vi "CommonVIs_SpltStringIntoArguments.vi"(1 "String":string="\"1,2,3\",120,\"pelle,12\"", 3 "AddEmptyValues(False)":bool, 5 "error in (no error)":errorcluster) -> (15 "splittedString":string[](array[string]), 19 "error out":errorcluster)   [LabVIEW 2020]
doc: "SubVI to a <B>ScriptText</B> object.\n\n[GOOP 1.0]"
panel:
  # "\"1,2,3\",120,\"pelle,12\""
  # "pelle,12"
  # "1,2,3"
  # "120"
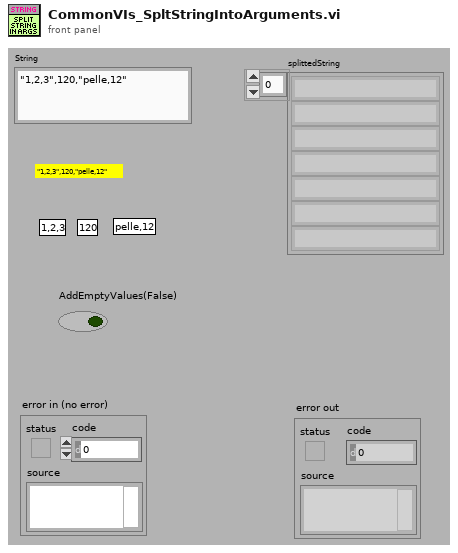
[diagram p1: front panel]
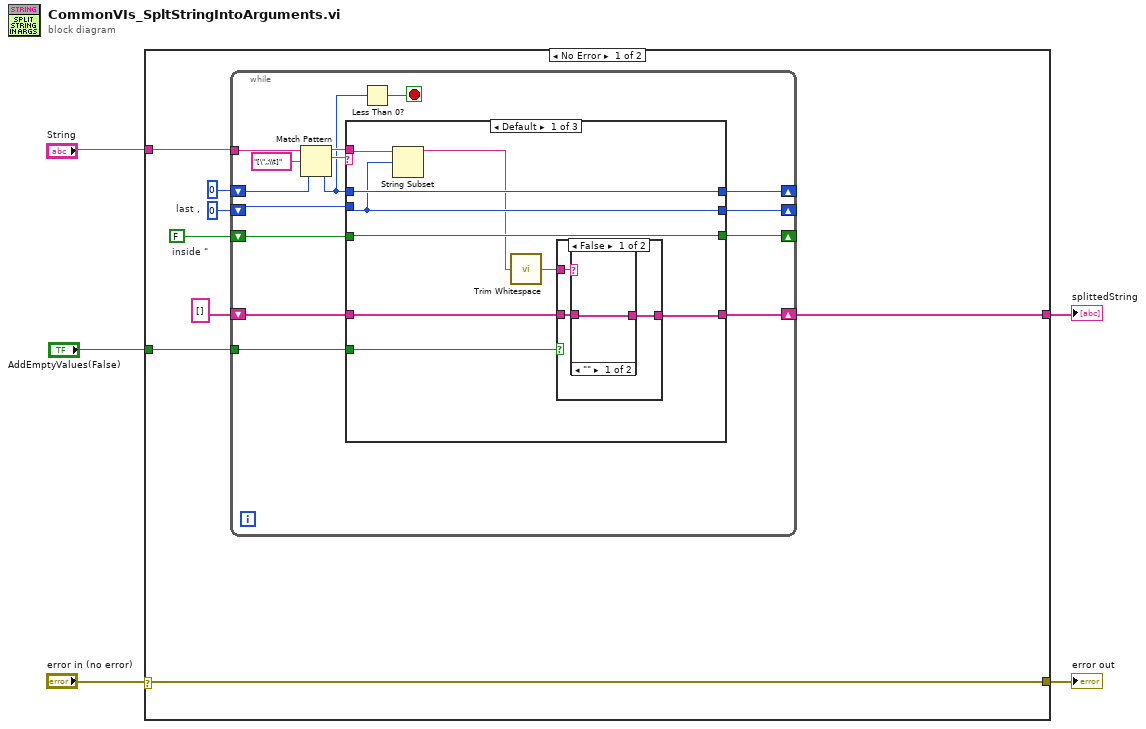
[diagram p0: block diagram]
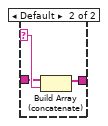
[diagram p2: hidden frame]
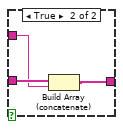
[diagram p3: hidden frame]
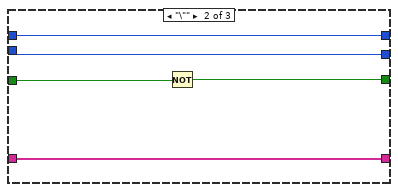
[diagram p4: hidden frame]
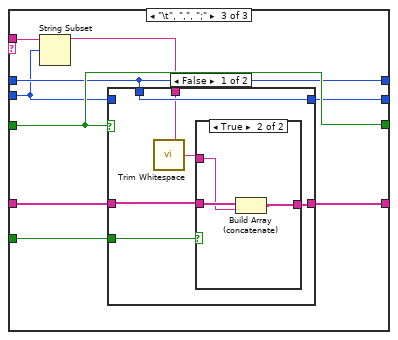
[diagram p5: hidden frame]
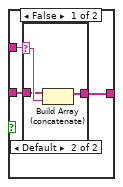
[diagram p6: hidden frame]
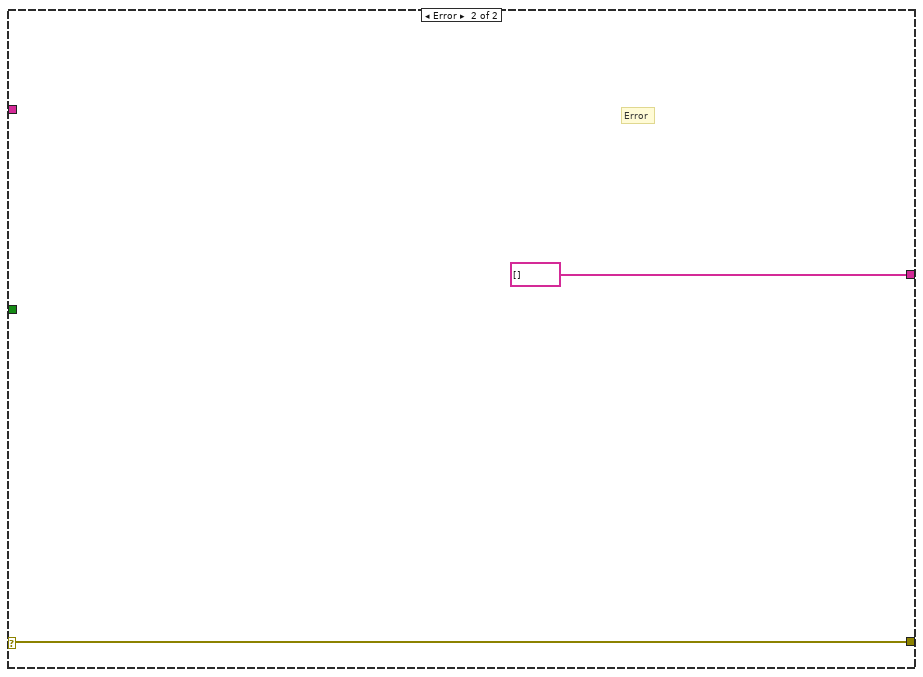
[diagram p9: hidden frame]
diagram:
  n1 = case shown="No Error" "error in (no error)" {
    selector: "error in (no error)" -> [w13 w81]
    tunnel: [w13 w81] -> w5
    tunnel: "String" -> [w12 _]
    tunnel: [w9 string[] [] ("splittedString")] -> w2
    tunnel: "AddEmptyValues(False)" -> [w6 _]
    frame No Error {
      w7 = 0  # last ,
      w8 = FALSE  # inside "
      n2 = while {
        shift-left: w7 -> [w16]
        shift-right: [w15] -> _
        shift-left: w8 -> [w25]
        shift-right: [w24] -> _
        shift-left: string[] [] ("splittedString") -> [w23]
        shift-right: [w22] -> w9
        shift-left: 0 -> [w17]
        shift-right: [w21] -> _
        tunnel: w12 -> [w27]
        tunnel: w6 -> [w14]
        stop <- w18 stop-if-true
        n3 = Match Pattern(string=w27, regular expression="[\",;\\t]", offset (0)=w17) -> (before substring=w20:string, match substring=w26:string, offset past match=w19:i32)  [unwired: 1 out]
        n4 = case shown="Default" w26 {
          tunnel: w25 -> [w36 w52 w60]
          tunnel: [w36 w51 w60] -> w24
          tunnel: w23 -> [w33 w50 w59]
          tunnel: [w32 w50 w61] -> w22
          tunnel: [w37 w49 w55] -> w21
          tunnel: w19 -> [w37 w49 w55]
          tunnel: w20 -> [w35 _ w58]
          tunnel: w16 -> [w34 w48 w54]
          tunnel: [w34 w48 w56] -> w15
          tunnel: w14 -> [w29 _ w53]
          frame Default {
            n5 = String Subset(string=w35, offset (0)=w34) -> (substring=w30:string)  [unwired: 1 out]
            n6 = call <vilib>:"Trim Whitespace.vi"("string"=w30) -> ("trimmed string"=w31:string)  [unwired: 1 in]
            n7 = case shown="False" w29 {
              tunnel: w33 -> [w40 w47]
              tunnel: [w39 w45] -> w32
              tunnel: w31 -> [w38 w46]
              frame False {
                n8 = case shown="\"\"" w38 {
                  selector: w38 -> [_ w44]
                  tunnel: [w41 w43] -> w39
                  tunnel: w40 -> [w41 w42]
                  frame "" {
                  }
                  frame Default {
                    n9 = Build Array (concatenate)(w42, w44) -> (w43:string[])
                  }
                }
              }
              frame True {
                n10 = Build Array (concatenate)(w47, w46) -> (w45:string[])
              }
            }
          }
          frame "\"" {
            n11 = Not(x=w52) -> (.not. x?=w51:bool)
          }
          frame "\t", ",", ";" {
            n12 = String Subset(string=w58, offset (0)=w54) -> (substring=w57:string)  [unwired: 1 out]
            n13 = case shown="False" w60 {
              tunnel: w59 -> [w64 w79]
              tunnel: [w62 w79] -> w61
              tunnel: w57 -> [w66 _]
              tunnel: [w67 w78] -> w56
              tunnel: w55 -> [w67 _]
              tunnel: w54 -> [_ w78]
              tunnel: w53 -> [w63 _]
              frame False {
                n14 = call <vilib>:"Trim Whitespace.vi"("string"=w66) -> ("trimmed string"=w65:string)  [unwired: 1 in]
                n15 = case shown="True" w63 {
                  tunnel: w64 -> [w70 w77]
                  tunnel: [w69 w75] -> w62
                  tunnel: w65 -> [w68 w76]
                  frame False {
                    n16 = case shown="Default" w68 {
                      selector: w68 -> [_ w74]
                      tunnel: [w71 w73] -> w69
                      tunnel: w70 -> [w71 w72]
                      frame "" {
                      }
                      frame Default {
                        n17 = Build Array (concatenate)(w72, w74) -> (w73:string[])
                      }
                    }
                  }
                  frame True {
                    n18 = Build Array (concatenate)(w77, w76) -> (w75:string[])
                  }
                }
              }
              frame True {
              }
            }
          }
        }
        n19 = Less Than 0?(x=w19) -> (x < 0?=w18:bool)
      }
    }
    frame Error {
      # "Error"
    }
  }
  "error out" <- w5
  "splittedString" <- w2
